vi "Analyze.vi"(8 "error in (no error)":errorcluster, 10 "Image in":T1, 11 "Analyze Q-Factor in":refnum<class "Analyze q-Factor.lvclass">) -> (0 "error out":errorcluster, 1 "Results":refnum<class "Analyze Results Base.lvclass">, 2 "Image out":T1, 3 "Analyze Q-Factor out":refnum<class "Analyze q-Factor.lvclass">)   [LabVIEW 2014, in "Analyze.lvlib" / "Analyze q-Factor.lvclass"]
uses:
  Analyze q-Factor.lvclass
  <vilib>/vision/Image Controls.llb/IMAQ Image.ctl
  Results and Overlays/Results Base/Analyze Results Base.lvclass
  Results and Overlays/Results q-Factor/Analyze Results q-Factor.lvclass
  Results and Overlays/Results Fluence/Analyze Results Fluence.lvclass
  Analyze Parameter/Analyze Parameter Width Method/Width Method.lvclass
  Results and Overlays/Results q-Factor/Analyze Results q-Factor.lvclass/Analyze Results q-Factor.ctl
  Results and Overlays/Results q-Factor/Write A.vi
  Results and Overlays/Results q-Factor/Write q.vi
  Results and Overlays/Results q-Factor/Write Focus ROI.vi
  Results and Overlays/Results q-Factor/Write Width Method.vi
  Analyze Fluence/Analyze Fluence.lvclass
  <vilib>/vision/NI_Vision_Development_Module.lvlib
  Analyze BaseClass/Analyze BaseClass/Analyze BaseClass.lvclass
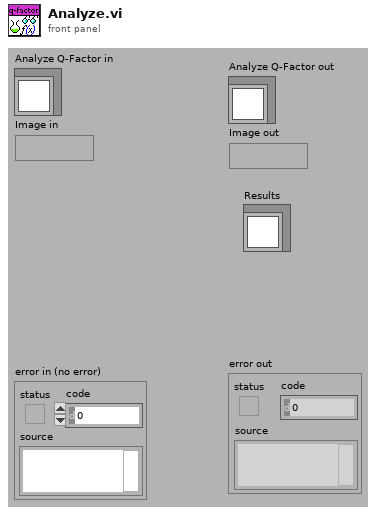
[diagram p1: front panel]
types:
  T1 = typedef "IMAQ Image.ctl" = refnum<image>
  T2 = typedef "Image Type" = u32
  T3 = typedef "Analyze.lvlib/Analyze Fluence.lvclass/Fluence Info.ctl" = cluster{"Fluence J/cm^2":dbl[unit], "Energy in Area":dbl[unit], "max value":i64, "Max fluence area":cluster{"Left":i32, "Top":i32, "Right":i32, "Bottom":i32}}
  T4 = cluster{"Left":i32, "Top":i32, "Right":i32, "Bottom":i32, sgl}
  T5 = typedef "POLARIS Vision utility.lvlib/Width Method.ctl" = enum16{"FWHM", "1/e", "1/e^2", "80%", "90%"}
  T6 = typedef "ROI Descriptor" = cluster{"Global Rectangle":i32[], "Contours":cluster{"ID":enum32{"External", "Internal"}, "Type":u32, "Coordinates":i32[]}[]}
  T7 = cluster{"Mean Value":sgl, "Standard Variation":sgl, "Minimal Value":sgl, "Maximal Value":sgl, "Area (calibrated)":sgl, "Area (pixels)":i32, "%":sgl}
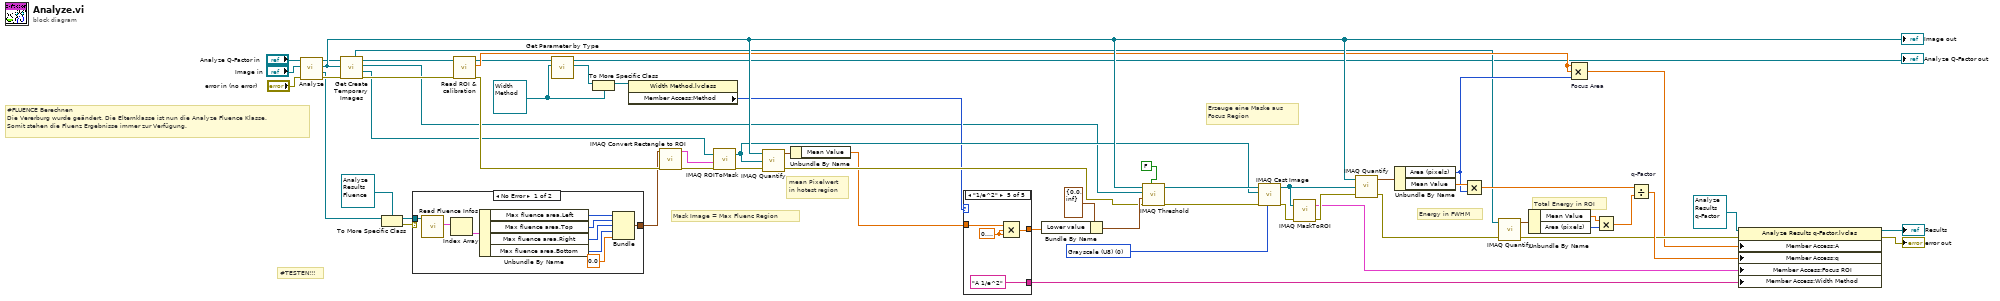
[diagram p0: block diagram]
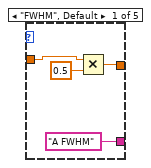
[diagram p3: hidden frame]
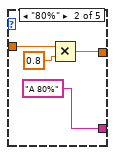
[diagram p4: hidden frame]
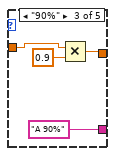
[diagram p5: hidden frame]
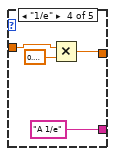
[diagram p6: hidden frame]
diagram:
  w2 = refnum<class "Width Method.lvclass"> refnum ("Width Method.lvclass")
  w53 = T2 0 items=["Grayscale (U8)", "Grayscale (I16)", "Grayscale (SGL)", "Complex (CSG)", "RGB (U32)", "HSL (U32)", "RGB (U64)", "Grayscale (U16)"] ("Image Type")
  # "#TESTEN!!!"
  # "Erzeuge eine Maske aus \nFocus Region"
  # "Mask Image = Max Fluenc Region"
  # "mean Pixelwert\nin hotest region"
  # "#FLUENCE Berechnen\nDie Vererburg wurde geändert. Die Elternklasse ist nun die Analyze Fluence Klasse.\nSomit stehen die Fluenz Ergebnisse immer zur Verfügung."
  # "Total Energy in ROI"
  # "Energy in FWHM"
  n1 = call-parent "Analyze.vi"("error in (no error)"="error in (no error)", "Image in"="Image in", "Analyze Fluence in"="Analyze Q-Factor in") -> ("error out"=w26:errorcluster, "Result"=w11:refnum<class "Analyze Results Base.lvclass">, "Image out"=w58:T1, "Analyze Fluence out"=w27:refnum<class "Analyze q-Factor.lvclass">)  [unwired: 5 in]
  "Image out" <- w58
  n2 = call-dynamic "Get Create Temporary Images.vi"("error in (no error)"=w26, "Image in"=w58, "Analyze BaseClass in"=w27) -> ("error out"=w33:errorcluster, "image mask"=w7:T1, "work image"=w5:T1, "Analyze BaseClass out"=w51:refnum<class "Analyze q-Factor.lvclass">, "masked image"=w6:T1)  [unwired: 4 in]
  n3 = To More Specific Class(target class=refnum<class "Analyze Results Fluence.lvclass"> refnum ("Analyze Results Fluence.lvclass"), reference=w11) -> (specific class reference=w10:refnum<class "Analyze Results Fluence.lvclass">, error out=w8:errorcluster)  [unwired: 1 in]
  n4 = case shown="No Error" w8 {
    tunnel: [w66 _] -> w17
    tunnel: w10 -> [w59 _]
    frame No Error {
      n5 = call-dynamic "Read Fluence Infos.vi"("Analyze Results Fluence in"=w59) -> ("Fluence Infos"=w61:T3[])  [unwired: 8 in, 2 out]
      n6 = Index Array(array=w61) -> (element=w60:T3)  [unwired: 1 in]
      n7 = Unbundle By Name(w60) -> ("Max fluence area.Left"=w65:i32, "Max fluence area.Top"=w64:i32, "Max fluence area.Right"=w63:i32, "Max fluence area.Bottom"=w62:i32)
      n8 = Bundle("Left"=w65, "Top"=w64, "Right"=w63, "Bottom"=w62, sgl 0.0) -> (w66:T4)  [unwired: 1 in]
    }
    frame Error {
    }
  }
  n9 = call-dynamic "Read ROI & calibration.vi"("error in (no error)"=w33, "Analyze BaseClass in"=w51) -> ("error out"=w32:errorcluster, "calibration mm/px"=w44:dbl[unit], "Analyze BaseClass out"=w12:refnum<class "Analyze q-Factor.lvclass">)  [unwired: 6 in, 1 out]
  n10 = call "Get Parameter by Type.vi"("Parameter Type"=w2, "Analyze BaseClass in"=w12) -> ("Parameter"=w3:refnum<class "Analyze Parameter Base.lvclass">, "Analyze BaseClass out"=→"Analyze Q-Factor out":refnum<class "Analyze q-Factor.lvclass">)  [unwired: 6 in, 2 out]
  n11 = To More Specific Class(target class=w2, reference=w3) -> (specific class reference=w1:refnum<class "Width Method.lvclass">)  [unwired: 1 in, 1 out]
  n12 = property class="Width Method.lvclass"(reference=w1) -> ("Member Access:Method"=w31:T5)  [unwired: 1 in, 2 out]
  n13 = call "IMAQ Convert Rectangle to ROI"("error in (no error)"=w32, "Rectangle"=w17) -> ("error out"=w15:errorcluster, "ROI Descriptor"=w16:T6)  [unwired: 7 in]
  n14 = call "IMAQ ROIToMask"("error in (no error)"=w15, "ROI Descriptor"=w16, "Image"=w7) -> ("error out"=w14:errorcluster, "Image Out"=w38:T1)  [unwired: 3 in, 1 out]
  n15 = call "IMAQ Quantify"("error in (no error)"=w14, "Image Mask"=w38, "Image"=w58) -> ("error out"=w37:errorcluster, "Global Report"=w13:T7)  [unwired: 1 out]
  n16 = Unbundle By Name(w13) -> ("Mean Value"=w36:sgl)
  n17 = case shown="\"1/e^2\"" w31 {
    tunnel: w36 -> [w70 w74 w78 w82 w87]
    tunnel: [w69 w73 w77 w81 w86] -> w45
    tunnel: ["A FWHM" "A 80%" "A 90%" "A 1/e" "A 1/e^2"] -> w23
    frame "FWHM", Default {
      n18 = Multiply(x=w70, y=0.5) -> (x*y=w69:dbl)
    }
    frame "80%" {
      n19 = Multiply(x=w74, y=0.8) -> (x*y=w73:dbl)
    }
    frame "90%" {
      n20 = Multiply(x=w78, y=0.9) -> (x*y=w77:dbl)
    }
    frame "1/e" {
      n21 = Multiply(x=w82, y=0.36787944117144233) -> (x*y=w81:dbl)
    }
    frame "1/e^2" {
      w85 = 0.36787944117144233
      n22 = Compound Arithmetic op=MULTIPLY(w87, w85, w85) -> (w86:dbl)
    }
  }
  n23 = Bundle By Name(cluster=cluster{"Lower value":sgl, "Upper value":sgl} {"Lower value"=0.0, "Upper value"=inf} ("Range"), "Lower value"=w45) -> (w56:cluster{"Lower value":sgl, "Upper value":sgl})
  n24 = call "IMAQ Threshold"("Keep/Replace Value (Replace)"=FALSE, "error in (no error)"=w37, "Range"=w56, "Image Dst"=w5, "Image Src"=w58) -> ("error out"=w54:errorcluster, "Image Dst Out"=w55:T1)  [unwired: 5 in]
  n25 = call "IMAQ Cast Image"("Image Type"=w53, "error in (no error)"=w54, "Image Dst"=w38, "Image Src"=w55) -> ("error out"=w40:errorcluster, "Image Dst Out"=w41:T1)  [unwired: 6 in]
  n26 = call "IMAQ MaskToROI"("Image"=w41, "error in (no error)"=w40) -> ("ROI Descriptor"=w22:T6, "error out"=w39:errorcluster)  [unwired: 5 in, 1 out]
  n27 = call "IMAQ Quantify"("error in (no error)"=w39, "Image Mask"=w41, "Image"=w58) -> ("error out"=w34:errorcluster, "Global Report"=w52:T7)  [unwired: 1 out]
  n28 = Unbundle By Name(w52) -> ("Area (pixels)"=w42:i32, "Mean Value"=w43:sgl)
  n29 = Multiply(x=w43, y=w42) -> (x*y=w46:sgl)
  n30 = call "IMAQ Quantify"("error in (no error)"=w34, "Image"=w6) -> ("error out"=w21:errorcluster, "Global Report"=w48:T7)  [unwired: 1 in, 1 out]
  n31 = Unbundle By Name(w48) -> ("Mean Value"=w50:sgl, "Area (pixels)"=w49:i32)
  n32 = Compound Arithmetic op=MULTIPLY "Focus Area"(w44, w44, w42) -> (w20:dbl[unit])
  n33 = Multiply(x=w50, y=w49) -> (x*y=w47:sgl)
  n34 = Divide "q-Factor"(x=w46, y=w47) -> (x/y=w24:sgl)
  n35 = property class="Analyze Results q-Factor.lvclas"(reference=refnum<class "Analyze Results q-Factor.lvclass"> refnum ("Analyze Results q-Factor.lvclass"), error in=w21, "Member Access:A"=w20, "Member Access:q"=w24, "Member Access:Focus ROI"=w22, "Member Access:Width Method"=w23) -> (reference out=→"Results":refnum<class "Analyze Results q-Factor.lvclass">, error out=→"error out":errorcluster)
